vi "读取.vi"(2 "命令":string, 3 "帧数":i32=2) -> (0 "error out":errorcluster, 1 "数组":string[](array[string]))   [LabVIEW 2014]
panel:
  in  "目标IP":string="192.168.0.2"
  in  "最大值(548)":i32=1024
  out "Actual Receive Buffer Size":u32
  in  "Set Receive Buffer Size(byte)":u32=64000000
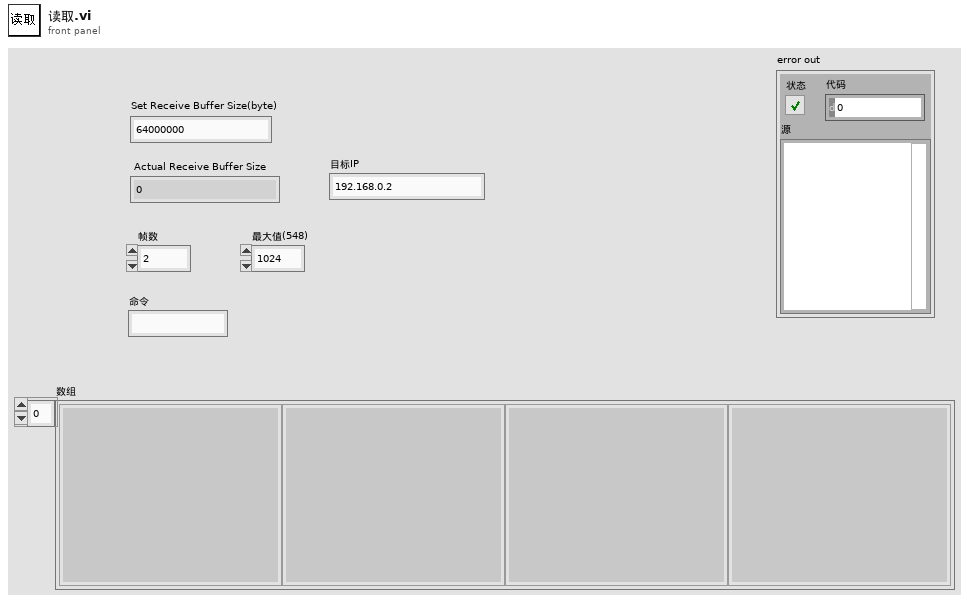
[diagram p1: front panel]
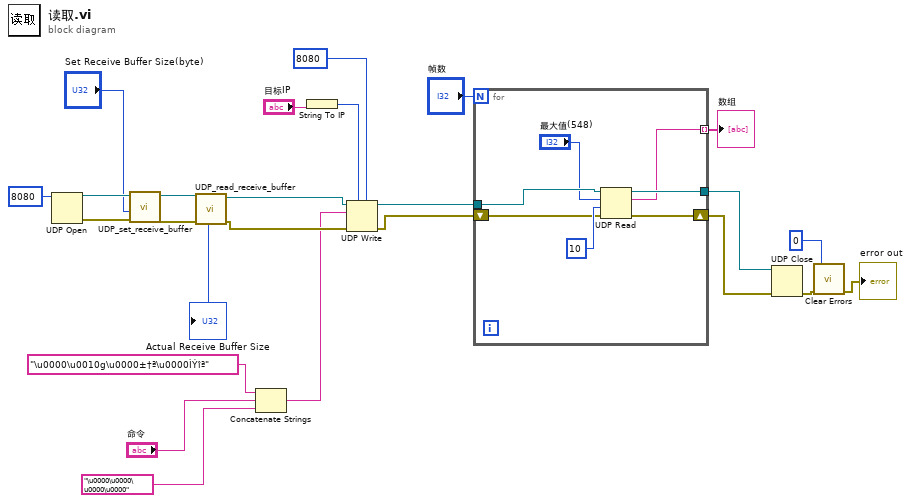
[diagram p0: block diagram]
diagram:
  n1 = UDP Open(11:u16 8080 ("端口")) -> (port=w22:refnum<k16>, 0:w21:errorcluster)  [unwired: 4 in, 1 out]
  n2 = call "UDP_set_receive_buffer.vi"("error in (no error)"=w21, "Receive Buffer Size"="Set Receive Buffer Size(byte)", "connection ID"=w22) -> ("error out"=w19:errorcluster, "connection ID out"=w20:refnum<k16>)  [unwired: 6 in]
  n3 = call "UDP_read_receive_buffer.vi"("error in (no error)"=w19, "connection ID"=w20) -> ("error out"=w16:errorcluster, "Receive Buffer Size"=→"Actual Receive Buffer Size":u32, "connection ID out"=w17:refnum<k16>)  [unwired: 5 in]
  n4 = Concatenate Strings("\u0000\u0010g\u0000±†ª\u0000ÌÝîª" ("字符串"), "命令", "\u0000\u0000\u0000\u0000" ("字符串")) -> (w6:string)
  n5 = String To IP(1:"目标IP") -> (0:w24:u32)
  n6 = UDP Write(address=w24, port or service name=u16 8080 ("端口或服务名称"), connection ID=w17, data in=w6, 8:w16) -> (error out=w14:errorcluster, 3:w15:refnum<k16>)  [unwired: 1 in]
  n7 = for {
    N: "帧数" -> [_]
    tunnel: w15 -> [w31]
    tunnel: [w29] -> w11
    tunnel: [w28] -> w9 mode=indexing
    shift-right: [w26] -> w7
    shift-left: w14 -> [w30]
    n8 = UDP Read(connection ID=w31, max size (548)="最大值(548)", timeout ms (25000)=10 ("超时毫秒(25000)"), 8:w30) -> (data out=w28:string, error out=w26:errorcluster, 3:w29:refnum<k16>)  [unwired: 2 out]
  }
  "数组" <- w9
  n9 = UDP Close(connection ID=w11, 8:w7) -> (error out=w13:errorcluster)  [unwired: 1 out]
  n10 = call <vilib>:"Clear Errors.vi"("error in (no error)"=w13, "specific error code to clear (0: all)"=0) -> ("error out"=→"error out":errorcluster)  [unwired: 4 in, 1 out]
